vi "Tutorial 05.vi"() -> ()   [LabVIEW 2014]
panel:
  out "Monthly Payment":dbl
  in  "Loan Amount":dbl
  in  "Months":dbl
  in  "Interest Rate":dbl
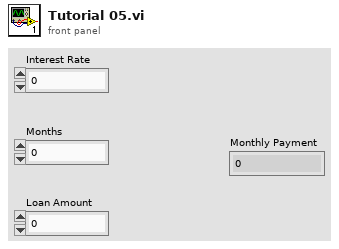
[diagram p1: front panel]
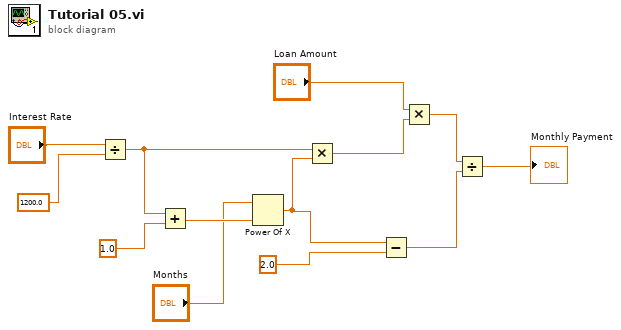
[diagram p0: block diagram]
diagram:
  n1 = Divide(x="Interest Rate", y=1200.0) -> (x/y=w11:dbl)
  n2 = Add(x=w11, y=1.0) -> (x+y=w9:dbl)
  n3 = Power Of X(1:w9, 2:"Months") -> (0:w7:dbl)
  n4 = Multiply(x=w11, y=w7) -> (x*y=w4:dbl)
  n5 = Subtract(x=w7, y=2.0) -> (x-y=w2:dbl)
  n6 = Multiply(x="Loan Amount", y=w4) -> (x*y=w3:dbl)
  n7 = Divide(x=w3, y=w2) -> (x/y=→"Monthly Payment":dbl)
